vi "open client handle.vi"(8 "error in (no error)":errorcluster, 10 "Request URI in":string, 11 "Oauth2 in":refnum<class "Oauth2.lvclass">) -> (0 "error out":errorcluster, 2 "Request URI dup":string, 3 "Oauth2 out":refnum<class "Oauth2.lvclass">)   [LabVIEW 2013, in "Oauth2.lvclass"]
uses:
  Oauth2.lvclass
  Oauth2.lvclass/Oauth2.ctl
  OauthClient/OAuthClient.lvclass
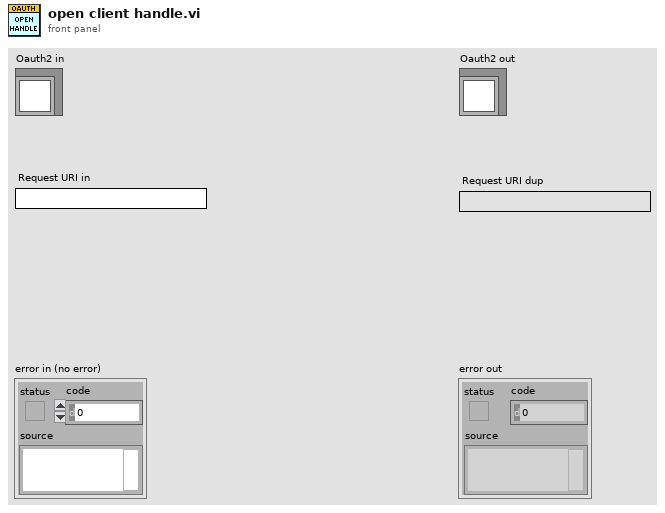
[diagram p1: front panel]
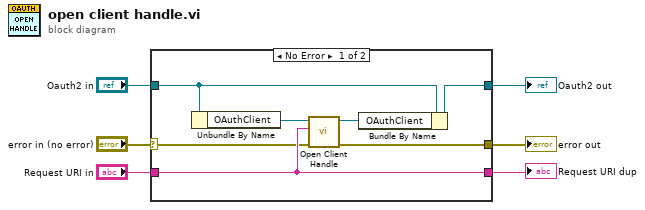
[diagram p0: block diagram]
diagram:
  n1 = case shown="No Error" "error in (no error)" {
    selector: "error in (no error)" -> [w11 w16]
    tunnel: [w10 w16] -> w5
    tunnel: [w7 w15] -> w3
    tunnel: "Oauth2 in" -> [w8 w15]
    tunnel: [w12 w14] -> w2
    tunnel: "Request URI in" -> [w12 w14]
    frame No Error {
      n2 = Unbundle By Name(w8) -> ("OAuthClient"=w13:refnum<class "OAuthClient.lvclass">)
      n3 = call-dynamic "Open Client Handle.vi"("error in (no error)"=w11, "Request URI"=w12, "OAuthClient in"=w13) -> ("error out"=w10:errorcluster, "OAuthClient out"=w9:refnum<class "OAuthClient.lvclass">)  [unwired: 7 in]
      n4 = Bundle By Name(cluster=w8, "OAuthClient"=w9) -> (w7:refnum<class "Oauth2.lvclass">)
    }
    frame Error {
    }
  }
  "error out" <- w5
  "Oauth2 out" <- w3
  "Request URI dup" <- w2
